vi "ResizeTreeCol1.vi"(8 "error in (no error)":errorcluster, 11 "TreeControl in":refnum<vi>) -> (0 "error out":errorcluster, 3 "TreeControl out":refnum<vi>)   [LabVIEW 2017]
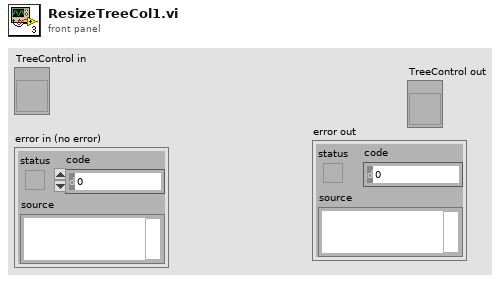
[diagram p1: front panel]
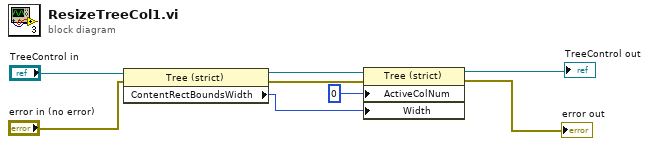
[diagram p0: block diagram]
diagram:
  n1 = property class="Tree (strict)"(reference="TreeControl in", error in="error in (no error)") -> (reference out=w6:refnum<vi>, error out=w5:errorcluster, "ContentRectBoundsWidth"=w3:i32)
  n2 = property class="Tree (strict)"(reference=w6, error in=w5, "ActiveColNum"=0 ("Active Cell:Active Column Number"), "Width"=w3) -> (reference out=→"TreeControl out":refnum<vi>, error out=→"error out":errorcluster)
